vi "Globals.vi"() -> ()   [LabVIEW 2017, in "NI_Robotics_Create Steering Frame.xnode"]
uses:
  <vilib>/robotics/Steering/Create Steering Frame/NI_Robotics_Create Steering Frame.xnode
panel:
  in  "Type Name":string="Configure Steering Frame"
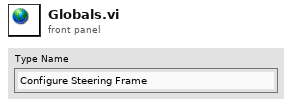
[diagram p1: front panel]
diagram:
